vi "digital_demod_host_sp_step_height_fb.vi"() -> ()   [LabVIEW 2018]
uses:
  <vilib>/userdefined/High Color/nirio_resource_hc.ctl
  <vilib>/LabVIEW Targets/FPGA/RIO/nirio_PxiTriggers.ctl
  <vilib>/UPVI/lvhdf5/file.llb/LVH5F Operation.ctl
  <vilib>/UPVI/lvhdf5/dataset.llb/LVH5D Operation.ctl
  <vilib>/Utility/miscctls.llb/LVRectTypeDef.ctl
  <vilib>/UPVI/lvhdf5/group.llb/H5G_obj_t.ctl
  <vilib>/FPGAPlugInAG/PXI-7854R/niLvFpga_Open_PXI-7854R.vi
  <vilib>/rvi/interface/common/dynamic/niFpgaDynamicAddResources.vi
  <vilib>/FPGAPlugInAG/Dynamic/niLvFpga_Run_Dynamic.vi
  <vilib>/LabVIEW Targets/FPGA/RIO/nirioReserveTrigger.vi
  <vilib>/Utility/error.llb/Error Cluster From Error Code.vi
  <vilib>/rvi/errors/niLvFpgaAdjustHostInterfaceError.vi
  <vilib>/UPVI/lvhdf5/utility.llb/Select HDF5 Dialog.vi
  <vilib>/UPVI/lvhdf5/utility.llb/Select HDF5 Dialog (Object Only).vi
  <vilib>/UPVI/lvhdf5/dataset.llb/Simple H5Dwrite (Variant).vi
  <vilib>/FPGAPlugInAG/Dynamic/niLvFpga_Close_Dynamic.vi
  <vilib>/rvi/interface/nirviOpenFPGA/nirviOpenFPGA.xnode
  FPGA Bitfiles/digitaldemod_FPGATarget_digitaldemodfpga_GFAocKRMO-I.lvbitx
  <vilib>/rvi/interface/nirviMethod/nirviMethod.xnode
  <vilib>/rvi/interface/nirviReadWriteControl/nirviReadWriteControl.xnode
  <vilib>/UPVI/lvhdf5/dataset.llb/Simple H5Dwrite.xnode
  <vilib>/UPVI/lvhdf5/library.llb/HDF5 Ref.ctl
  <vilib>/rvi/interface/nirviCloseFPGA/nirviCloseFPGA.xnode
  <vilib>/rvi/interface/Simulation/niFpgaSimulationCallBeginRW.vi
  <vilib>/rvi/errors/niLvFpgaMergeErrorWithErrorCode.vi
  <vilib>/FPGAPlugInAG/Dynamic/niLvFpga_ReadFifo_Dynamic.vi
  NiFpgaLv.dll
  <vilib>/FPGAPlugInAG/Dynamic/niLvFpga_StartFifo_Dynamic.vi
  <vilib>/FPGAPlugInAG/Dynamic/niLvFpga_StopFifo_Dynamic.vi
  FPGA Timekeeper 1.1b0/FPGA Timekeeper.lvlib
  <vilib>/UPVI/lvhdf5/identifier.llb/Not an HDF5 Refnum Constant.vi
  <vilib>/UPVI/lvhdf5/dataset.llb/OpenCreateReplace Dataset by Element Type.vi
  <vilib>/UPVI/lvhdf5/dataspace.llb/H5Sselect_hyperslab.vi
  <vilib>/UPVI/lvhdf5/dataset.llb/H5Dwrite (Variant).vi
  <vilib>/UPVI/lvhdf5/dataset.llb/H5Dget_space.vi
  <vilib>/UPVI/lvhdf5/attribute.llb/private/LVH5AwriteWDTAttrs.vi
  <vilib>/UPVI/lvhdf5/dataspace.llb/H5Sclose.vi
  <vilib>/UPVI/lvhdf5/dataset.llb/H5Dclose.vi
  <vilib>/UPVI/lvhdf5/utility.llb/Select HDF5 Dialog (File and Object).vi
panel:
  in  "z_set_min":dbl=-920000.0
  in  "z_set_max":dbl=-850000.0
  out "current_z_set":dbl=-850500.0
  in  "step_lower_lim":dbl=-5000.0
  in  "step_upper_lim":dbl=5000.0
  out "height_fb":dbl=1600.0
  in  "height_pg":dbl=-10000.0
  in  "height_set_point":dbl=-0.8
  in  "Counts per update":i32=10000
  in  "Height_fb_counter":i32=7860
  in  "Height feedback":bool
  in  "Height_pcc":dbl=0.05
  in  "subtract_zfb_ndelay":u8=1
  in  "subtract_zfb_delay":bool=TRUE
  out "pow_fb":i16(graph)=-50
  in  "subtract_zfb_i_scale":fxp<+/-,32,16>=-17.0
  in  "subtract_zfb_p_scale":fxp<+/-,32,16>=-23.0
  in  "subtract_zfb_d_scale":fxp<+/-,32,16>=-13.0
  in  "subtract_zfb_from_powerr":bool=TRUE
  in  "sum_z-pow_fb":bool=TRUE
  in  "delta_pow_set_llim":fxp<+/-,32,32>=-80000.0
  in  "delta_pow_set_ulim":fxp<+/-,32,32>=80000.0
  in  "fb_on_powset":bool
  in  "pow_lower_lim":i16=-2000
  in  "pow_upper_lim":i16=2000
  in  "pow_dc_offset":i16=-17200
  in  "pow_dg":fxp<+/-,32,16>
  in  "pow_pg":fxp<+/-,32,16>
  in  "pow_fb":bool=TRUE
  out "pow_set_actual":fxp<+/-,33,33>=-34500.0
  in  "reset_pow_accum":bool
  in  "pow_bitshift":i16=-6
  in  "pow_fb_bitshift":i16=-16
  in  "pow_ig":fxp<+/-,32,16>=0.00140380859375
  in  "pow_set_user":fxp<+/-,32,32>=-34500.0
  out "pow":i32(graph)=-37680
  out "delta_pow_set":dbl(graph)
  in  "DAQ_trig":bool
  in  "save_data":bool=TRUE
  out "z_fb_tot":i16(graph)=-17096
  in  "z_off_restart":bool
  in  "z_off_step":i16=-17500
  in  "z_off_start":i16=-17500
  in  "step_z_offset":bool
  in  "z_set_step":fxp<+/-,32,32>
  in  "step_z_set":bool
  out "z_set_user":fxp<+/-,32,32>=-860000.0
  in  "set_z_init":bool
  in  "reset_zphi_and_change":bool
  in  "reset_z_accum":bool
  in  "z_lower_lim":i16=-3000
  in  "z_upper_lim":i16=3000
  in  "z_fb_bitshift":i16=-16
  in  "z_ig":fxp<+/-,32,16>=-1.52587890625e-05
  in  "z_dg":fxp<+/-,32,16>=-0.205291748046875
  in  "z_pg":fxp<+/-,32,16>=-0.010528564453125
  in  "z_bitshift":i16
  in  "z_set_init":fxp<+/-,32,32>=-860000.0
  in  "z_dc_offset":i16
  in  "z_internal_inject_scale":i16=400
  in  "z_internal_inject_freq":fxp<+,32,0>=2.00001522898674e-05 format="%#_32g"
  in  "add_sin":bool
  in  "show_quad":bool=TRUE
  out "delta_phi":cluster{dbl, dbl, dbl, dbl}(graph)={0.0, 0.05572509765625, 0.1119384765625, 0.0279541015625}
  in  "xy2_bitshift":i16
  in  "xy_fb_bitshift":i16=-16
  in  "y_lower_lim":i16=-1000
  in  "y_upper_lim":i16=1000
  in  "y_dg":fxp<+/-,32,16>=-0.004974365234375
  in  "x_lower_lim":i16=-1000
  in  "x_upper_lim":i16=1000
  in  "x_dg":fxp<+/-,32,16>=0.004974365234375
  in  "xy_bitshift":i16=-10
  in  "y_dc_offset":i16
  in  "x_dc_offset":i16
  in  "downsample->xyz":bool
  in  "inject_sigs":bool
  in  "Load last pars":bool
  out "config_trig":bool
  in  "block_hardware_trigs":bool
  out "config_loaded":bool
  out "Nsamp_config":u32=40000
  out "fpga_dat_path":path=path "D:/data/20210329/bead2/turbombar_powfb_xyzcool_1_fpga.h5"
  in  "reset_trigs":bool
  in  "accept_trigs":bool=TRUE
  out "amp4":dbl(graph)=9833.655883789062
  out "phi4":dbl(graph)=-66.42401123046875
  in  "Change Pars 2":bool
  out "z_fb":i16(graph)=154
  out "z":i32(graph)=-850000
  out "y_fb":i16(graph)=3
  out "y":i32(graph)=-88958
  out "x_fb":i16(graph)
  out "x":i32(graph)=-3908
  out "Host time (ns)":u64=1617643596633207808
  out "Target time (ns)":u64=1617643596633246868
  in  "downsamp_num":i16=100
  in  "Reset Phi Params":T1={"All Phi?"=FALSE, "Which?"=enum."3"}
  out "amp2":dbl(graph)=4850.323699951172
  out "amp3":dbl(graph)=5487.453506469727
  out "amp0":dbl(graph)=5014.9466552734375
  out "amp1":dbl(graph)=5412.640853881836
  out "phi2":dbl(graph)=-6.08233642578125
  out "phi3":dbl(graph)=-6.16632080078125
  in  "subtract_mean":bool=TRUE
  out "loop time":fxp<+,32,32>=2.0
  in  "Change Pars":bool
  out "phi0":dbl(graph)=-6.19427490234375
  out "phi1":dbl(graph)=-6.1385498046875
  in  "counter offset":u32
  in  "phase discont_neg":fxp<+/-,24,12>=-1.0
  in  "phase discont_pos":fxp<+/-,24,12>=1.0
  in  "Reset Phi":bool
  in  "loop timer (usec)":u32=2
  in  "Update ADC Clock":bool
  in  "Host Update Rate (msec)":dbl=1.0 format="%#_13g"
  in  "RIO Device":T2="RIO0"
  # "QPD AMPLITUDES"
  # "QPD PHASES"
  # "BACKSCATTER"
  # "BEAD XYZ + FB"
  # "FEEDBACK NESTING"
  # "Height feedback"
  # "POWER FEEDBACK"
  # "Z FEEDBACK"
  # "X FEEDBACK"
  # "Y FEEDBACK"
types:
  T1 = cluster{"All Phi?":bool, "Which?":enum16{"0", "1", "2", "3", "4"}}
  T2 = typedef "nirio_resource_hc.ctl" = tag
  T3 = typedef "nirio_PxiTriggers.ctl" = u16
  T4 = cluster{"phase discont_pos":fxp<+/-,24,12>, "phase discont_neg":fxp<+/-,24,12>, "counter offset":u32, "subtract_mean":bool, "downsamp_num":i16, "xy_bitshift":i16, "x_dg":fxp<+/-,32,16>, "x_upper_lim":i16, "x_lower_lim":i16, "x_dc_offset":i16, "y_dg":fxp<+/-,32,16>, "y_upper_lim":i16, "y_lower_lim":i16, "y_dc_offset":i16, "xy_fb_bitshift":i16, "z_bitshift":i16, "z_set_init":fxp<+/-,32,32>, "z_pg":fxp<+/-,32,16>, "z_dg":fxp<+/-,32,16>, "z_ig":fxp<+/-,32,16>, "z_fb_bitshift":i16, "z_upper_lim":i16, "z_lower_lim":i16, "z_off_start":i16, "inject_sigs":bool, "downsample->xyz":bool, "xy2_bitshift":i16, "add_sin":bool, "z_internal_inject_freq":fxp<+,32,0>, "z_internal_inject_scale":i16, "pow_bitshift":i16, "pow_set_user":fxp<+/-,32,32>, "pow_pg":fxp<+/-,32,16>, "pow_dg":fxp<+/-,32,16>, "pow_ig":fxp<+/-,32,16>, "pow_dc_offset":i16, "pow_upper_lim":i16, "pow_lower_lim":i16, "pow_fb_bitshift":i16, "pow_fb":bool, "fb_on_powset":bool, "delta_pow_set_ulim":fxp<+/-,32,32>, "delta_pow_set_llim":fxp<+/-,32,32>, "sum_z-pow_fb":bool, "subtract_zfb_from_powerr":bool, "subtract_zfb_p_scale":fxp<+/-,32,16>, "subtract_zfb_i_scale":fxp<+/-,32,16>, "subtract_zfb_d_scale":fxp<+/-,32,16>, "subtract_zfb_delay":bool, "subtract_zfb_ndelay":u8}
  T5 = enum16{"open", "replace", "create", "open or create", "replace or create", "replace or create with confirmation"}
  T6 = typedef "LVH5F Operation.ctl" = enum16{"open", "open or create", "create or replace", "create or replace (with confirmation)", "create", "open (read only)"}
  T7 = typedef "LVRectTypeDef.ctl" = cluster{"Left":i16, "Top":i16, "Right":i16, "Bottom":i16}
  T8 = cluster{"Behavior":enum32{"Invalid", "Default", "Floating", "Floating/Auto-Hide", "Modal"}, "Position":T7, "Center":bool, "Title":string}
  T9 = typedef "LVH5D Operation.ctl" = enum16{"open", "replace", "create", "open or create", "create or replace", "create or replace with confirmation"}
  T10 = typedef "H5G_obj_t.ctl" = i32
  T11 = cluster{"Object Types (any)":T10[], "Object Pattern":string}
  T12 = typedef "HDF5 Ref.ctl" = refnum<k1>
  T13 = cluster{fxp<+/-,33,19>, fxp<+/-,33,19>, fxp<+/-,33,19>, fxp<+/-,33,19>}
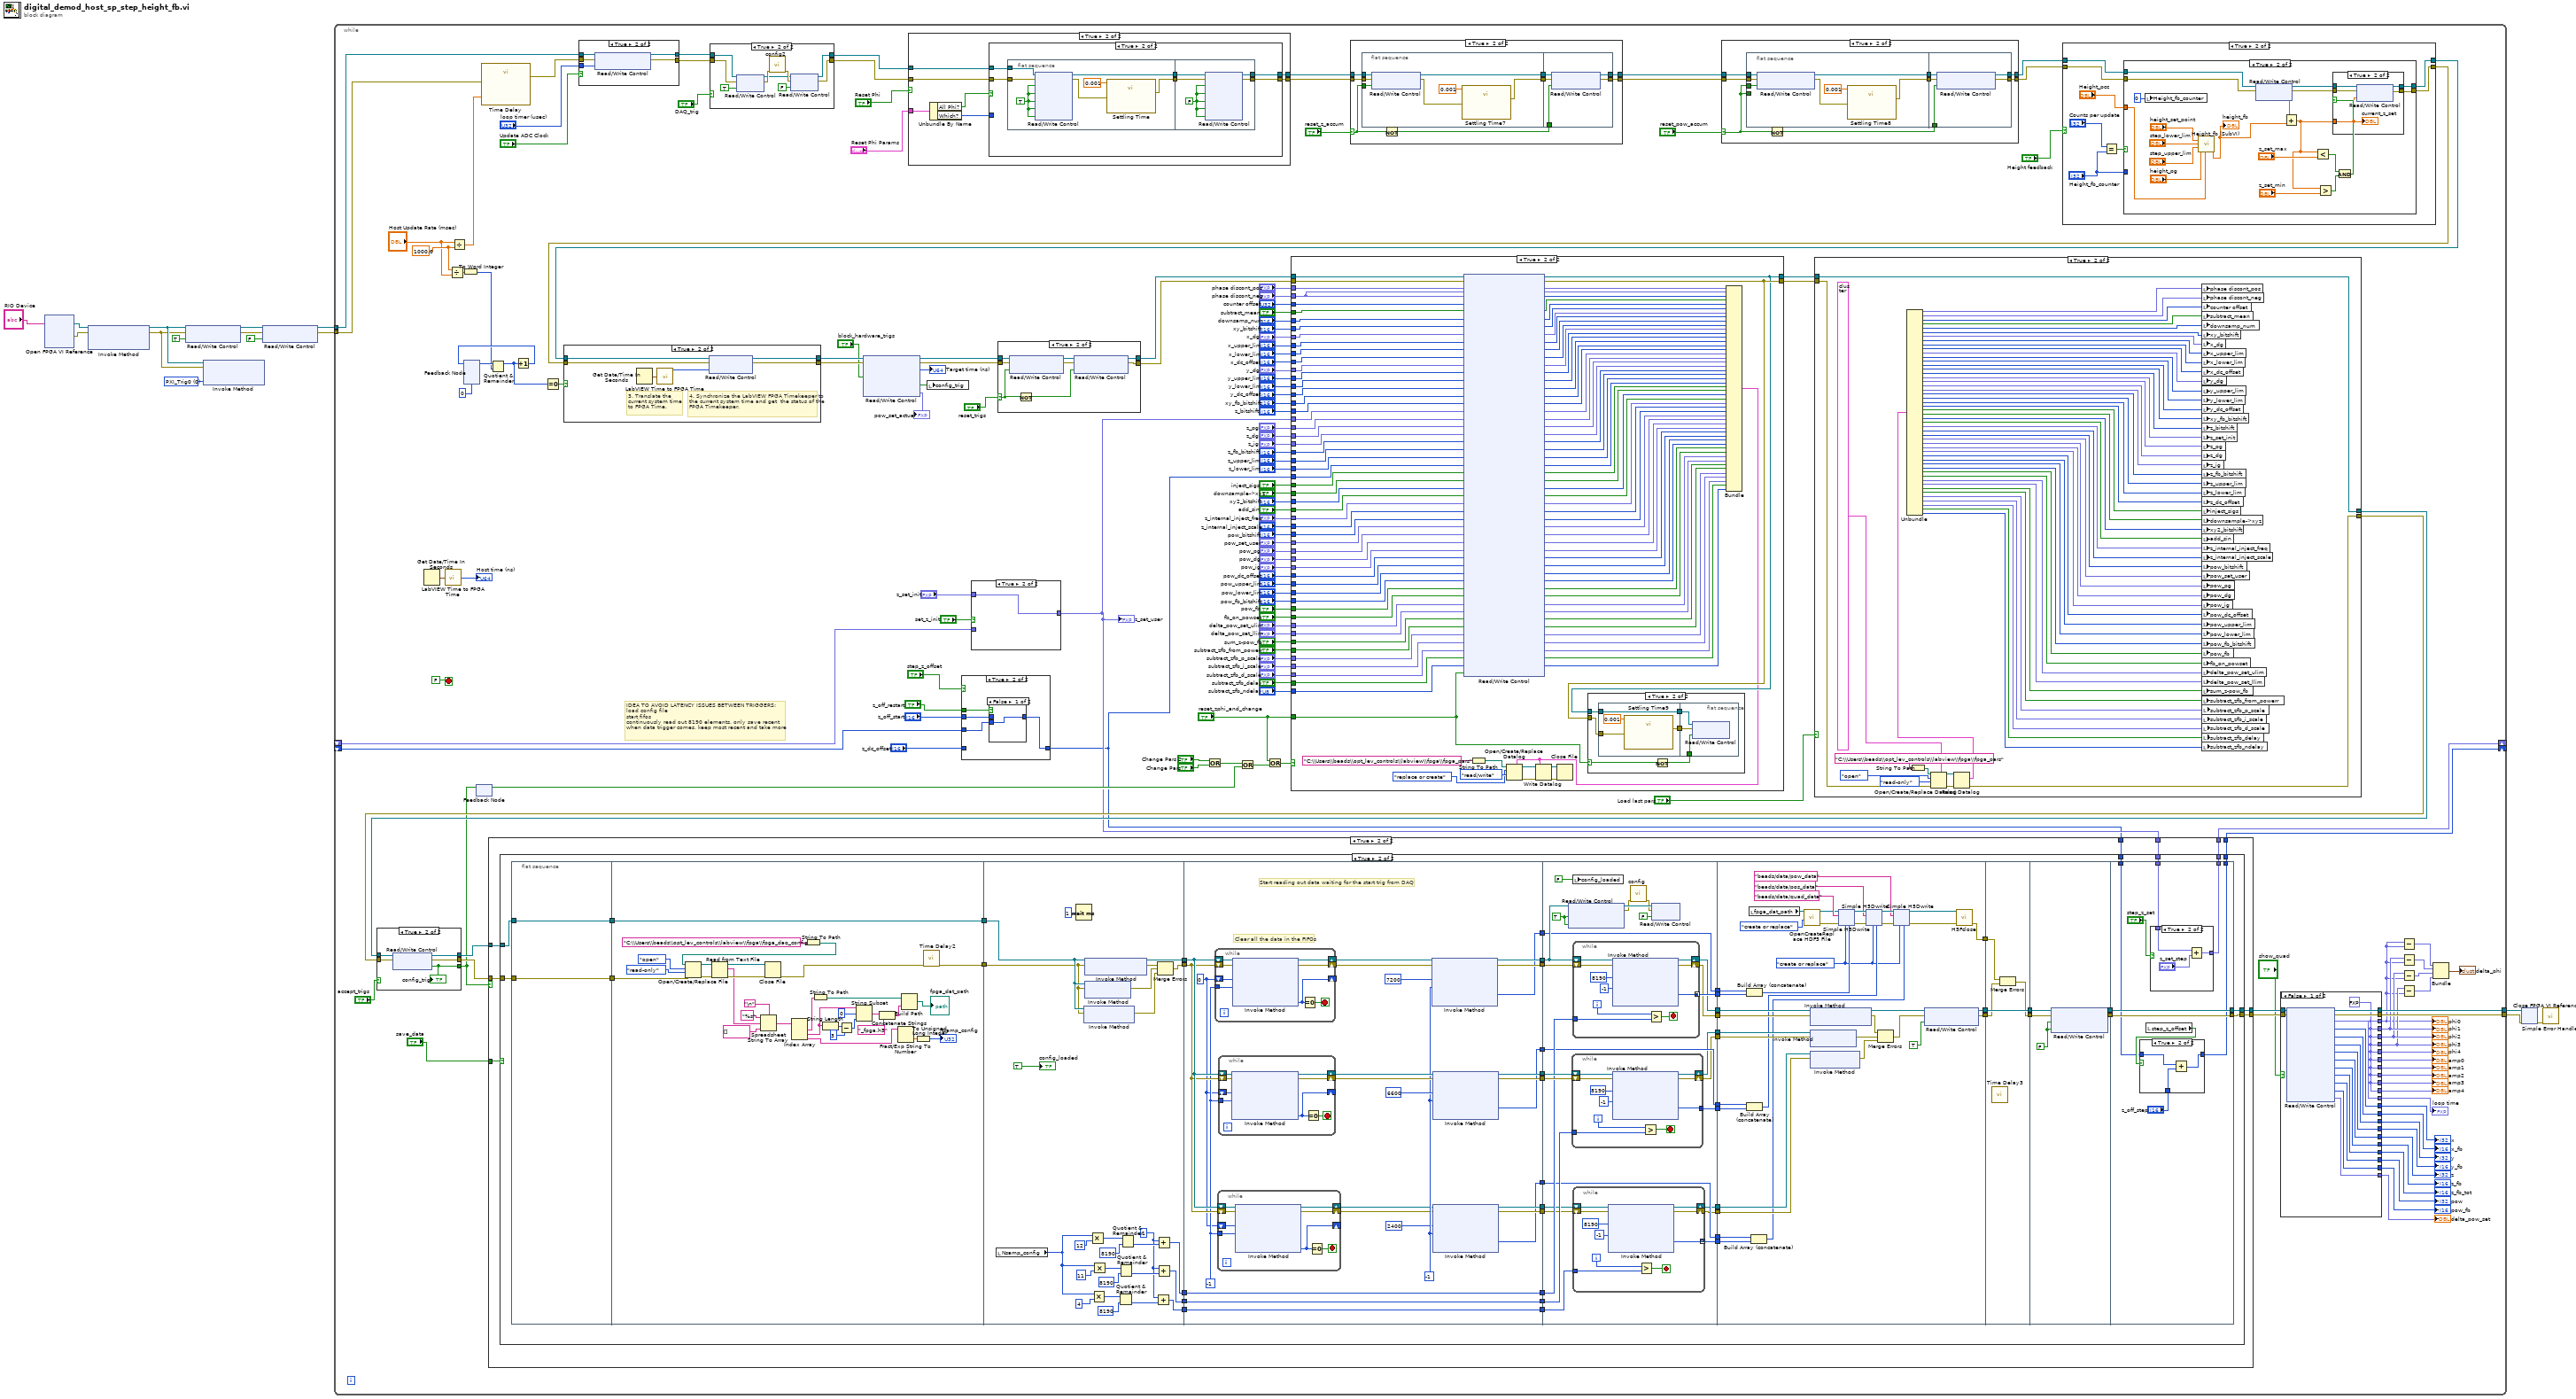
[diagram p0: block diagram]
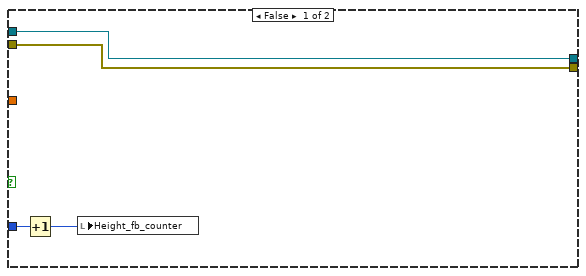
[diagram p3: hidden frame]
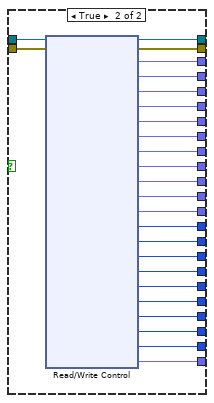
[diagram p10: hidden frame]
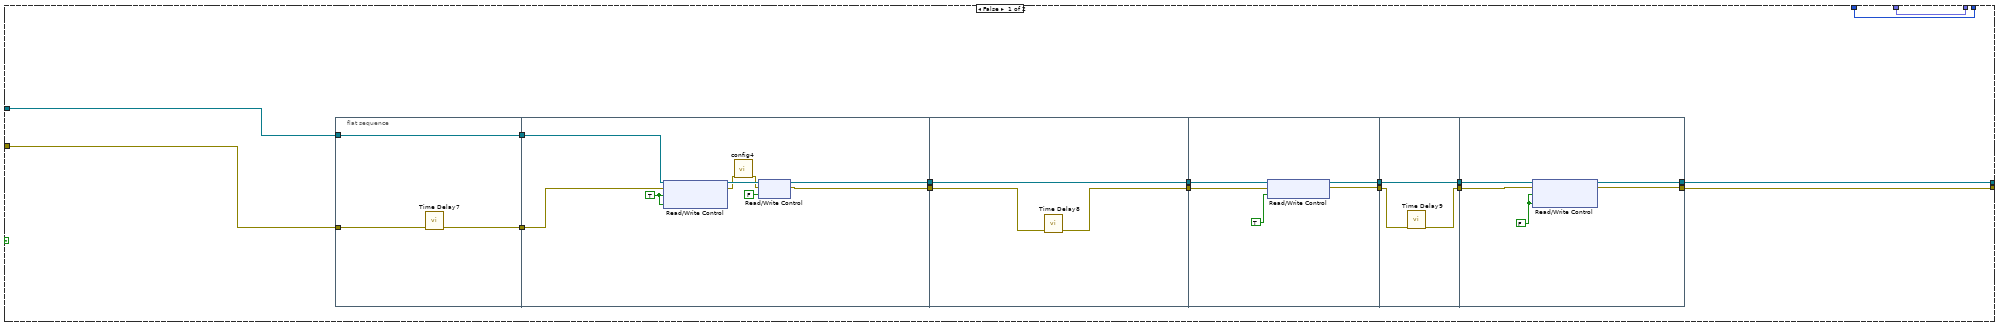
[diagram p15: hidden frame]
diagram:
  w1 = T3 0 items=["PXI_Trig0", "PXI_Trig1", "PXI_Trig2", "PXI_Trig3", "PXI_Trig4", "PXI_Trig5", "PXI_Trig6", "PXI_Trig7"] ("Trigger")
  n1 = xnode "Open FPGA VI Reference"("resource name"="RIO Device") -> ("FPGA VI Reference Out"=w11:refnum<k20>, "error out"=w10:errorcluster)  [unwired: 1 in]
  n2 = xnode "Invoke Method"("FPGA VI Reference In"=w11, "error in"=w10) -> ("FPGA VI Reference Out"=w3:refnum<k20>, "error out"=w2:errorcluster)  [unwired: 1 in]
  n3 = xnode "Read/Write Control"("FPGA VI Reference In"=w3, "error in"=w2, "reset_config_trig"=TRUE ("reset_trig")) -> ("FPGA VI Reference Out"=w6:refnum<k20>, "error out"=w4:errorcluster)
  n4 = xnode "Invoke Method"("FPGA VI Reference In"=w3, "error in"=w2, "Trigger"=w1) -> ()  [unwired: 2 out]
  n5 = xnode "Read/Write Control"("FPGA VI Reference In"=w6, "error in"=w4, "reset_config_trig"=FALSE ("manual_trig")) -> ("FPGA VI Reference Out"=w9:refnum<k20>, "error out"=w8:errorcluster)
  n6 = while {
    tunnel: w8 -> [w169]
    tunnel: w9 -> [w95]
    tunnel: [w162] -> w14
    tunnel: [w161] -> w13
    shift-right: [w73] -> _
    shift-left: _ -> [w74]
    shift-right: [w65] -> _
    shift-left: _ -> [w64]
    stop <- FALSE stop-if-true
    w152 = 1000.0
    # "IDEA TO AVOID LATENCY ISSUES BETWEEN TRIGGERS:\nload config file\nstart fifos\ncontinuously read out 8190 elements, only save recent\nwhen data trigger comes, keep most recent and take more"
    n7 = Get Date/Time In Seconds() -> (seconds since 1Jan1904=w141:timestamp)
    n8 = call "LabVIEW Time to FPGA Time.vi"("LabVIEW time"=w141) -> ("FPGA time (ns)"=→"Host time (ns)":u64)
    n9 = Divide(x=w152, y="Host Update Rate (msec)") -> (x/y=w150:dbl)
    n10 = Divide(x="Host Update Rate (msec)", y=w152) -> (x/y=w170:dbl)
    n11 = To Word Integer(number=w150) -> (16bit integer=w144:i16)
    n12 = feedback #1(i16 0) -> (w146:i16)
    n13 = feedback #2() -> (w76:bool)  [unwired: 1 in]
    n14 = call "Time Delay"("error in (no error)"=w169, "Delay Time (s)"=w170) -> ("error out"=w167:errorcluster)  [unwired: 9 in]
    n15 = Quotient & Remainder(x=w146, y=w144) -> (x-y*floor(x/y)=w143:i16)  [unwired: 1 out]
    n16 = Increment(x=w143) -> (x+1=w145:i16)
    n17 = feedback-in #1(w145) -> ()
    n18 = Equal To 0?(x=w143) -> (x = 0?=w148:bool)
    n19 = case shown="True" "Update ADC Clock" {
      tunnel: w95 -> [w1549 w1554]
      tunnel: w167 -> [w1548 w1553]
      tunnel: [w1549 w1552] -> w53
      tunnel: [w1548 w1551] -> w52
      tunnel: "loop timer (usec)" -> [_ w1550]
      frame False {
      }
      frame True {
        n20 = xnode "Read/Write Control"("FPGA VI Reference In"=w1554, "error in"=w1553, "loop timer (usec)"=w1550) -> ("FPGA VI Reference Out"=w1552:refnum<k20>, "error out"=w1551:errorcluster)
      }
    }
    n21 = case shown="True" "DAQ_trig" {
      tunnel: w53 -> [w235 w239]
      tunnel: w52 -> [w234 w238]
      tunnel: [w235 w237] -> w51
      tunnel: [w234 w236] -> w50
      frame False {
      }
      frame True {
        n22 = xnode "Read/Write Control"("FPGA VI Reference In"=w239, "error in"=w238, "TRIG0"=TRUE) -> ("FPGA VI Reference Out"=w241:refnum<k20>, "error out"=w242:errorcluster)
        n23 = call "config2"("error in (no error)"=w242) -> ("error out"=w243:errorcluster)  [unwired: 10 in]
        n24 = xnode "Read/Write Control"("FPGA VI Reference In"=w241, "error in"=w243, "TRIG0"=FALSE) -> ("FPGA VI Reference Out"=w237:refnum<k20>, "error out"=w236:errorcluster)
      }
    }
    n25 = case shown="True" "Reset Phi" {
      tunnel: w51 -> [w1427 w1434]
      tunnel: w50 -> [w1426 w1433]
      tunnel: [w1427 w1431] -> w99
      tunnel: [w1426 w1432] -> w98
      tunnel: "Reset Phi Params" -> [_ w1430]
      frame False {
      }
      frame True {
        n26 = Unbundle By Name(w1430) -> ("All Phi?"=w1429:bool, "Which?"=w1428:enum16{"0", "1", "2", "3", "4"})
        n27 = case shown="True" w1429 {
          tunnel: w1434 -> [w1439 w1533]
          tunnel: w1433 -> [w1438 w1532]
          tunnel: [w1436 w1531] -> w1432
          tunnel: [w1437 w1530] -> w1431
          tunnel: w1428 -> [w1435 _]
          frame False {
            n28 = case shown="\"4\"" w1435 {
              tunnel: w1439 -> [w1443 w1461 w1479 w1497 w1515]
              tunnel: w1438 -> [w1442 w1460 w1478 w1496 w1514]
              tunnel: [w1441 w1459 w1477 w1495 w1513] -> w1437
              tunnel: [w1440 w1458 w1476 w1494 w1512] -> w1436
              frame "1" {
                n29 = flat-sequence {
                  tunnel: w1443 -> [w1452]
                  tunnel: w1442 -> [w1451]
                  tunnel: [w1450] -> w1445
                  tunnel: [w1447] -> w1444
                  tunnel: w1445 -> [w1457]
                  tunnel: w1444 -> [w1456]
                  tunnel: [w1455] -> w1441
                  tunnel: [w1454] -> w1440
                  frame #0 {
                    n30 = xnode "Read/Write Control"("FPGA VI Reference In"=w1452, "error in"=w1451, "reset_phi1"=TRUE) -> ("FPGA VI Reference Out"=w1450:refnum<k20>, "error out"=w1448:errorcluster)
                    n31 = call "Settling Time2"("error in (no error)"=w1448, "Delay Time (s)"=0.001) -> ("error out"=w1447:errorcluster)  [unwired: 9 in]
                  }
                  frame #1 {
                    n32 = xnode "Read/Write Control"("FPGA VI Reference In"=w1457, "error in"=w1456, "reset_phi1"=FALSE) -> ("FPGA VI Reference Out"=w1455:refnum<k20>, "error out"=w1454:errorcluster)
                  }
                }
              }
              frame "2" {
                n33 = flat-sequence {
                  tunnel: w1461 -> [w1470]
                  tunnel: w1460 -> [w1469]
                  tunnel: [w1468] -> w1463
                  tunnel: [w1465] -> w1462
                  tunnel: w1463 -> [w1475]
                  tunnel: w1462 -> [w1474]
                  tunnel: [w1473] -> w1459
                  tunnel: [w1472] -> w1458
                  frame #0 {
                    n34 = xnode "Read/Write Control"("FPGA VI Reference In"=w1470, "error in"=w1469, "reset_phi2"=TRUE) -> ("FPGA VI Reference Out"=w1468:refnum<k20>, "error out"=w1466:errorcluster)
                    n35 = call "Settling Time3"("error in (no error)"=w1466, "Delay Time (s)"=0.001) -> ("error out"=w1465:errorcluster)  [unwired: 9 in]
                  }
                  frame #1 {
                    n36 = xnode "Read/Write Control"("FPGA VI Reference In"=w1475, "error in"=w1474, "reset_phi2"=FALSE) -> ("FPGA VI Reference Out"=w1473:refnum<k20>, "error out"=w1472:errorcluster)
                  }
                }
              }
              frame "3" {
                n37 = flat-sequence {
                  tunnel: w1479 -> [w1488]
                  tunnel: w1478 -> [w1487]
                  tunnel: [w1486] -> w1481
                  tunnel: [w1483] -> w1480
                  tunnel: w1481 -> [w1493]
                  tunnel: w1480 -> [w1492]
                  tunnel: [w1491] -> w1477
                  tunnel: [w1490] -> w1476
                  frame #0 {
                    n38 = xnode "Read/Write Control"("FPGA VI Reference In"=w1488, "error in"=w1487, "reset_phi3"=TRUE) -> ("FPGA VI Reference Out"=w1486:refnum<k20>, "error out"=w1484:errorcluster)
                    n39 = call "Settling Time4"("error in (no error)"=w1484, "Delay Time (s)"=0.001) -> ("error out"=w1483:errorcluster)  [unwired: 9 in]
                  }
                  frame #1 {
                    n40 = xnode "Read/Write Control"("FPGA VI Reference In"=w1493, "error in"=w1492, "reset_phi3"=FALSE) -> ("FPGA VI Reference Out"=w1491:refnum<k20>, "error out"=w1490:errorcluster)
                  }
                }
              }
              frame "4" {
                n41 = flat-sequence {
                  tunnel: w1497 -> [w1506]
                  tunnel: w1496 -> [w1505]
                  tunnel: [w1504] -> w1499
                  tunnel: [w1501] -> w1498
                  tunnel: w1499 -> [w1511]
                  tunnel: w1498 -> [w1510]
                  tunnel: [w1509] -> w1495
                  tunnel: [w1508] -> w1494
                  frame #0 {
                    n42 = xnode "Read/Write Control"("FPGA VI Reference In"=w1506, "error in"=w1505, "reset_phi4"=TRUE) -> ("FPGA VI Reference Out"=w1504:refnum<k20>, "error out"=w1502:errorcluster)
                    n43 = call "Settling Time5"("error in (no error)"=w1502, "Delay Time (s)"=0.001) -> ("error out"=w1501:errorcluster)  [unwired: 9 in]
                  }
                  frame #1 {
                    n44 = xnode "Read/Write Control"("FPGA VI Reference In"=w1511, "error in"=w1510, "reset_phi4"=FALSE) -> ("FPGA VI Reference Out"=w1509:refnum<k20>, "error out"=w1508:errorcluster)
                  }
                }
              }
              frame "0" {
                n45 = flat-sequence {
                  tunnel: w1515 -> [w1524]
                  tunnel: w1514 -> [w1523]
                  tunnel: [w1522] -> w1517
                  tunnel: [w1519] -> w1516
                  tunnel: w1517 -> [w1529]
                  tunnel: w1516 -> [w1528]
                  tunnel: [w1527] -> w1513
                  tunnel: [w1526] -> w1512
                  frame #0 {
                    n46 = xnode "Read/Write Control"("FPGA VI Reference In"=w1524, "error in"=w1523, "reset_phi0"=TRUE) -> ("FPGA VI Reference Out"=w1522:refnum<k20>, "error out"=w1520:errorcluster)
                    n47 = call "Settling Time6"("error in (no error)"=w1520, "Delay Time (s)"=0.001) -> ("error out"=w1519:errorcluster)  [unwired: 9 in]
                  }
                  frame #1 {
                    n48 = xnode "Read/Write Control"("FPGA VI Reference In"=w1529, "error in"=w1528, "reset_phi0"=FALSE) -> ("FPGA VI Reference Out"=w1527:refnum<k20>, "error out"=w1526:errorcluster)
                  }
                }
              }
            }
          }
          frame True {
            n49 = flat-sequence {
              tunnel: w1533 -> [w1542]
              tunnel: w1532 -> [w1541]
              tunnel: [w1540] -> w1535
              tunnel: [w1537] -> w1534
              tunnel: w1535 -> [w1547]
              tunnel: w1534 -> [w1546]
              tunnel: [w1545] -> w1530
              tunnel: [w1544] -> w1531
              frame #0 {
                w1536 = TRUE
                n50 = xnode "Read/Write Control"("FPGA VI Reference In"=w1542, "error in"=w1541, "reset_phi0"=w1536, "reset_phi1"=w1536, "reset_phi2"=w1536, "reset_phi3"=w1536, "reset_phi4"=w1536) -> ("FPGA VI Reference Out"=w1540:refnum<k20>, "error out"=w1538:errorcluster)
                n51 = call "Settling Time"("error in (no error)"=w1538, "Delay Time (s)"=0.001) -> ("error out"=w1537:errorcluster)  [unwired: 9 in]
              }
              frame #1 {
                w1543 = FALSE
                n52 = xnode "Read/Write Control"("FPGA VI Reference In"=w1547, "error in"=w1546, "reset_phi0"=w1543, "reset_phi1"=w1543, "reset_phi2"=w1543, "reset_phi3"=w1543, "reset_phi4"=w1543) -> ("FPGA VI Reference Out"=w1545:refnum<k20>, "error out"=w1544:errorcluster)
              }
            }
          }
        }
      }
    }
    n53 = case shown="True" "step_z_offset" {
      tunnel: [w245 w246] -> w66
      tunnel: "z_dc_offset" -> [w245 _]
      tunnel: w64 -> [_ w248]
      tunnel: "z_off_start" -> [_ w249]
      tunnel: "z_off_restart" -> [_ w247]
      frame False {
      }
      frame True {
        n54 = case shown="False" w247 {
          tunnel: w249 -> [_ w251]
          tunnel: w248 -> [w250 _]
          tunnel: [w250 w251] -> w246
          frame False {
          }
          frame True {
          }
        }
      }
    }
    n55 = case shown="True" "set_z_init" {
      tunnel: [w252 w253] -> w72
      tunnel: "z_set_init" -> [_ w253]
      tunnel: w74 -> [w252 _]
      frame False {
      }
      frame True {
      }
    }
    "z_set_user" <- w72
    n56 = Or(x="Change Pars 2", y="Change Pars") -> (x .or. y?=w29:bool)
    n57 = Or(x=w29, y=w76) -> (x .or. y?=w27:bool)
    n58 = Or(x="reset_zphi_and_change", y=w27) -> (x .or. y?=w26:bool)
    n59 = case shown="True" "reset_z_accum" {
      selector: "reset_z_accum" -> [_ w361]
      tunnel: w99 -> [w359 w367]
      tunnel: w98 -> [w358 w366]
      tunnel: [w359 w365] -> w49
      tunnel: [w358 w364] -> w48
      frame False {
      }
      frame True {
        n60 = flat-sequence {
          tunnel: w367 -> [w374]
          tunnel: w366 -> [w373]
          tunnel: w361 -> [w371]
          tunnel: [w372] -> w363
          tunnel: [w368] -> w362
          tunnel: [w376] -> w364
          tunnel: [w377] -> w365
          tunnel: w363 -> [w379]
          tunnel: w362 -> [w378]
          tunnel: w360 -> [w375]
          frame #0 {
            n61 = xnode "Read/Write Control"("FPGA VI Reference In"=w374, "error in"=w373, "reset_z_accum"=w371) -> ("FPGA VI Reference Out"=w372:refnum<k20>, "error out"=w369:errorcluster)
            n62 = call "Settling Time7"("error in (no error)"=w369, "Delay Time (s)"=0.001) -> ("error out"=w368:errorcluster)  [unwired: 9 in]
          }
          frame #1 {
            n63 = xnode "Read/Write Control"("FPGA VI Reference In"=w379, "error in"=w378, "reset_z_accum"=w375) -> ("FPGA VI Reference Out"=w377:refnum<k20>, "error out"=w376:errorcluster)
          }
        }
        n64 = Not(x=w361) -> (.not. x?=w360:bool)
      }
    }
    n65 = case shown="True" "reset_pow_accum" {
      selector: "reset_pow_accum" -> [_ w216]
      tunnel: w49 -> [w213 w218]
      tunnel: w48 -> [w212 w217]
      tunnel: [w213 w215] -> w19
      tunnel: [w212 w214] -> w17
      frame False {
      }
      frame True {
        n66 = flat-sequence {
          tunnel: w218 -> [w228]
          tunnel: w217 -> [w227]
          tunnel: w216 -> [w225]
          tunnel: [w226] -> w221
          tunnel: [w222] -> w220
          tunnel: w216 -> [_]
          tunnel: [w229] -> _
          tunnel: [w231] -> w215
          tunnel: w221 -> [w233]
          tunnel: w220 -> [w232]
          tunnel: w219 -> [w230]
          tunnel: [w229] -> w214
          frame #0 {
            n67 = xnode "Read/Write Control"("FPGA VI Reference In"=w228, "error in"=w227, "reset_pow_accum"=w225) -> ("FPGA VI Reference Out"=w226:refnum<k20>, "error out"=w223:errorcluster)
            n68 = call "Settling Time8"("error in (no error)"=w223, "Delay Time (s)"=0.001) -> ("error out"=w222:errorcluster)  [unwired: 9 in]
          }
          frame #1 {
            n69 = xnode "Read/Write Control"("FPGA VI Reference In"=w233, "error in"=w232, "reset_pow_accum"=w230) -> ("FPGA VI Reference Out"=w231:refnum<k20>, "error out"=w229:errorcluster)
          }
        }
        n70 = Not(x=w216) -> (.not. x?=w219:bool)
      }
    }
    n71 = case shown="True" "Height feedback" {
      tunnel: w19 -> [w172 w175]
      tunnel: [w172 w173] -> w18
      tunnel: w17 -> [w171 w176]
      tunnel: [w171 w174] -> w16
      frame False {
      }
      frame True {
        n72 = Equal?(x="Counts per update", y="Height_fb_counter") -> (x = y?=w180:bool)
        n73 = case shown="True" w180 {
          tunnel: "Height_fb_counter" -> [w183 _]
          tunnel: "Height_pcc" -> [_ w203]
          tunnel: w176 -> [w181 w197]
          tunnel: w175 -> [w182 w198]
          tunnel: [w181 w196] -> w174
          tunnel: [w182 w195] -> w173
          frame False {
            n74 = Increment(x=w183) -> (x+1=w184:i32)
            n75 = local write "Height_fb_counter"(w184) -> ()
          }
          frame True {
            n76 = local write "Height_fb_counter"(0 ("Height_fb_counter")) -> ()
            n77 = call "Height_fb (SubVI).vi"("Height_pcc"=w203, "height_set_point"="height_set_point", "height_pg"="height_pg", "step_upper_lim"="step_upper_lim", "step_lower_lim"="step_lower_lim") -> ("hieght_fb_out"=w191:dbl)  [unwired: 5 in, 1 out]
            "height_fb" <- w191
            n78 = xnode "Read/Write Control"("FPGA VI Reference In"=w198, "error in"=w197) -> ("FPGA VI Reference Out"=w194:refnum<k20>, "error out"=w193:errorcluster, "z_set_user"=w192:fxp<+/-,32,32>)
            n79 = Add(x=w192, y=w191) -> (x+y=w186:dbl)
            n80 = Less?(x=w186, y="z_set_max") -> (x < y?=w187:bool)
            n81 = Greater?(x=w186, y="z_set_min") -> (0:w188:bool)
            n82 = And(x=w187, y=w188) -> (x .and. y?=w185:bool)
            n83 = case shown="True" w185 {
              tunnel: [w205 w211] -> w196
              tunnel: [w206 w210] -> w195
              tunnel: w194 -> [w206 w209]
              tunnel: w193 -> [w205 w208]
              tunnel: w186 -> [_ w207]
              frame False {
              }
              frame True {
                n84 = xnode "Read/Write Control"("FPGA VI Reference In"=w209, "error in"=w208, "z_set_user"=w207) -> ("FPGA VI Reference Out"=w210:refnum<k20>, "error out"=w211:errorcluster)
                "current_z_set" <- w207
              }
            }
          }
        }
      }
    }
    n85 = case shown="True" w148 {
      tunnel: w16 -> [w1339 w1344]
      tunnel: w18 -> [w1340 w1343]
      tunnel: [w1340 w1342] -> w139
      tunnel: [w1339 w1341] -> w138
      frame False {
      }
      frame True {
        # "4. Synchronize the LabVIEW FPGA Timekeeper to the current system time and get  the status of the FPGA Timekeeper."
        # "3. Translate the current system time to FPGA Time."
        n86 = Get Date/Time In Seconds() -> (seconds since 1Jan1904=w1346:timestamp)
        n87 = call "LabVIEW Time to FPGA Time.vi"("LabVIEW time"=w1346) -> ("FPGA time (ns)"=w1345:u64)
        n88 = xnode "Read/Write Control"("FPGA VI Reference In"=w1343, "error in"=w1344, "RT time (ns)"=w1345) -> ("FPGA VI Reference Out"=w1342:refnum<k20>, "error out"=w1341:errorcluster)
      }
    }
    n89 = xnode "Read/Write Control"("FPGA VI Reference In"=w139, "error in"=w138, "block_config_trig"="block_hardware_trigs") -> ("FPGA VI Reference Out"=w110:refnum<k20>, "error out"=w109:errorcluster, "time (ns)"=→"Target time (ns)":u64, "config_trig"=w96:bool, "pow_set_actual"=→"pow_set_actual":fxp<+/-,33,33>)
    n90 = local write "config_trig"(w96) -> ()
    n91 = case shown="True" "reset_trigs" {
      selector: "reset_trigs" -> [_ w1332]
      tunnel: w110 -> [w1330 w1338]
      tunnel: w109 -> [w1329 w1337]
      tunnel: [w1330 w1334] -> w106
      tunnel: [w1329 w1333] -> w105
      frame False {
      }
      frame True {
        n92 = xnode "Read/Write Control"("FPGA VI Reference In"=w1338, "error in"=w1337, "reset_config_trig"=w1332) -> ("FPGA VI Reference Out"=w1336:refnum<k20>, "error out"=w1335:errorcluster)
        n93 = Not(x=w1332) -> (.not. x?=w1331:bool)
        n94 = xnode "Read/Write Control"("FPGA VI Reference In"=w1336, "error in"=w1335, "reset_config_trig"=w1331) -> ("FPGA VI Reference Out"=w1334:refnum<k20>, "error out"=w1333:errorcluster)
      }
    }
    n95 = case shown="True" w26 {
      tunnel: w105 -> [w1348 w1411]
      tunnel: [w1348 w1354] -> w92
      tunnel: [w1347 w1353] -> w94
      tunnel: w106 -> [w1347 w1412]
      tunnel: "phase discont_pos" -> [_ w1410]
      tunnel: "phase discont_neg" -> [_ w1409]
      tunnel: "counter offset" -> [_ w1408]
      tunnel: "subtract_mean" -> [_ w1407]
      tunnel: "downsamp_num" -> [_ w1406]
      tunnel: "x_dc_offset" -> [_ w1401]
      tunnel: "y_dc_offset" -> [_ w1397]
      tunnel: w66 -> [_ w1387]
      tunnel: w72 -> [_ w1394]
      tunnel: "xy_bitshift" -> [_ w1405]
      tunnel: "x_dg" -> [_ w1404]
      tunnel: "x_upper_lim" -> [_ w1403]
      tunnel: "x_lower_lim" -> [_ w1402]
      tunnel: "y_dg" -> [_ w1400]
      tunnel: "y_upper_lim" -> [_ w1399]
      tunnel: "y_lower_lim" -> [_ w1398]
      tunnel: "z_bitshift" -> [_ w1395]
      tunnel: "z_pg" -> [_ w1393]
      tunnel: "z_dg" -> [_ w1392]
      tunnel: "z_ig" -> [_ w1391]
      tunnel: "z_fb_bitshift" -> [_ w1390]
      tunnel: "z_upper_lim" -> [_ w1389]
      tunnel: "z_lower_lim" -> [_ w1388]
      tunnel: "xy_fb_bitshift" -> [_ w1396]
      tunnel: "inject_sigs" -> [_ w1378]
      tunnel: "downsample->xyz" -> [_ w1377]
      tunnel: "xy2_bitshift" -> [_ w1376]
      tunnel: "add_sin" -> [_ w1375]
      tunnel: "z_internal_inject_freq" -> [_ w1374]
      tunnel: "z_internal_inject_scale" -> [_ w1373]
      tunnel: "pow_set_user" -> [_ w1371]
      tunnel: "pow_ig" -> [_ w1370]
      tunnel: "pow_fb_bitshift" -> [_ w1364]
      tunnel: "pow_bitshift" -> [_ w1372]
      tunnel: "fb_on_powset" -> [_ w1362]
      tunnel: "delta_pow_set_ulim" -> [_ w1361]
      tunnel: "delta_pow_set_llim" -> [_ w1360]
      tunnel: "pow_fb" -> [_ w1363]
      tunnel: "pow_pg" -> [_ w1368]
      tunnel: "pow_dg" -> [_ w1369]
      tunnel: "pow_dc_offset" -> [_ w1367]
      tunnel: "pow_upper_lim" -> [_ w1366]
      tunnel: "pow_lower_lim" -> [_ w1365]
      tunnel: "sum_z-pow_fb" -> [_ w1359]
      tunnel: "subtract_zfb_from_powerr" -> [_ w1358]
      tunnel: "subtract_zfb_d_scale" -> [_ w1357]
      tunnel: "subtract_zfb_p_scale" -> [_ w1356]
      tunnel: "subtract_zfb_i_scale" -> [_ w1355]
      tunnel: "reset_zphi_and_change" -> [_ w1351]
      tunnel: "subtract_zfb_delay" -> [_ w1350]
      tunnel: "subtract_zfb_ndelay" -> [_ w1349]
      frame False {
      }
      frame True {
        n96 = xnode "Read/Write Control"("FPGA VI Reference In"=w1412, "error in"=w1411, "discont_pos"=w1410, "discont_neg"=w1409, "Counter Offset"=w1408, "subtract_mean"=w1407, "downsamp_num"=w1406, "xy_bitshift"=w1405, "x_dg"=w1404, "x_upper_lim"=w1403, "x_lower_lim"=w1402, "x_dc_offset"=w1401, "y_dg"=w1400, "y_upper_lim"=w1399, "y_lower_lim"=w1398, "y_dc_offset"=w1397, "xy_fb_bitshift"=w1396, "z_bitshift"=w1395, "z_set_user"=w1394, "z_pg"=w1393, "z_dg"=w1392, "z_ig"=w1391, "z_fb_bitshift"=w1390, "z_upper_lim"=w1389, "z_lower_lim"=w1388, "z_dc_offset"=w1387, "inject_sigs"=w1378, "downsample->xyz"=w1377, "xy2_bitshift"=w1376, "add_sin"=w1375, "z_internal_inject_freq"=w1374, "z_internal_inject_scale"=w1373, "pow_bitshift"=w1372, "pow_set_user"=w1371, "pow_pg"=w1368, "pow_dg"=w1369, "pow_ig"=w1370, "pow_dc_offset"=w1367, "pow_upper_lim"=w1366, "pow_lower_lim"=w1365, "pow_fb_bitshift"=w1364, "pow_fb"=w1363, "fb_on_pow_set"=w1362, "delta_pow_set_ulim"=w1361, "delta_pow_set_llim"=w1360, "sum_z-pow_fb"=w1359, "subtract_zfb_from_powerr"=w1358, "subtract_zfb_p_scale"=w1356, "subtract_zfb_i_scale"=w1355, "subtract_zfb_d_scale"=w1357, "subtract_zfb_delay"=w1350, "subtract_zfb_ndelay"=w1349, "reset_phi4"=w1351) -> ("FPGA VI Reference Out"=w1353:refnum<k20>, "error out"=w1354:errorcluster)
        n97 = String To Path(string="C:\\Users\\beads\\opt_lev_controls\\labview\\fpga\\fpga_pars") -> (path=w1380:path)
        n98 = case shown="True" w1351 {
          selector: w1351 -> [_ w1414]
          tunnel: w1354 -> [_ w1416]
          tunnel: w1353 -> [_ w1417]
          frame False {
          }
          frame True {
            n99 = flat-sequence {
              tunnel: [w1421] -> w1418
              tunnel: w1417 -> [w1421]
              tunnel: w1416 -> [w1420]
              tunnel: [w1419] -> w1415
              tunnel: w1418 -> [w1425]
              tunnel: w1415 -> [w1424]
              tunnel: w1413 -> [w1423]
              frame #0 {
                n100 = call "Settling Time9"("error in (no error)"=w1420, "Delay Time (s)"=0.001) -> ("error out"=w1419:errorcluster)  [unwired: 9 in]
              }
              frame #1 {
                n101 = xnode "Read/Write Control"("FPGA VI Reference In"=w1425, "error in"=w1424, "reset_phi4"=w1423) -> ()  [unwired: 2 out]
              }
            }
            n102 = Not(x=w1414) -> (.not. x?=w1413:bool)
          }
        }
        n103 = Bundle("phase discont_pos"=w1410, "phase discont_neg"=w1409, "counter offset"=w1408, "subtract_mean"=w1407, "downsamp_num"=w1406, "xy_bitshift"=w1405, "x_dg"=w1404, "x_upper_lim"=w1403, "x_lower_lim"=w1402, "x_dc_offset"=w1401, "y_dg"=w1400, "y_upper_lim"=w1399, "y_lower_lim"=w1398, "y_dc_offset"=w1397, "xy_fb_bitshift"=w1396, "z_bitshift"=w1395, "z_set_init"=w1394, "z_pg"=w1393, "z_dg"=w1392, "z_ig"=w1391, "z_fb_bitshift"=w1390, "z_upper_lim"=w1389, "z_lower_lim"=w1388, "z_off_start"=w1387, "inject_sigs"=w1378, "downsample->xyz"=w1377, "xy2_bitshift"=w1376, "add_sin"=w1375, "z_internal_inject_freq"=w1374, "z_internal_inject_scale"=w1373, "pow_bitshift"=w1372, "pow_set_user"=w1371, "pow_pg"=w1368, "pow_dg"=w1369, "pow_ig"=w1370, "pow_dc_offset"=w1367, "pow_upper_lim"=w1366, "pow_lower_lim"=w1365, "pow_fb_bitshift"=w1364, "pow_fb"=w1363, "fb_on_powset"=w1362, "delta_pow_set_ulim"=w1361, "delta_pow_set_llim"=w1360, "sum_z-pow_fb"=w1359, "subtract_zfb_from_powerr"=w1358, "subtract_zfb_p_scale"=w1356, "subtract_zfb_i_scale"=w1355, "subtract_zfb_d_scale"=w1357, "subtract_zfb_delay"=w1350, "subtract_zfb_ndelay"=w1349) -> (w1352:T4)  [unwired: 1 in]
        n104 = Open/Create/Replace Datalog(5:w1352, 9:enum16{"read/write", "read-only", "write-only"}."read/write" ("access (0:read/write)"), 10:T5."replace or create" ("operation (0:open)"), 11:w1380) -> (0:w1386:errorcluster, 3:w1384:refnum<k1>)  [unwired: 2 in, 1 out]
        n105 = Write Datalog(4:w1386, 6:w1352, 7:w1384) -> (0:w1385:errorcluster, 3:w1383:refnum<k1>)
        n106 = Close File(refnum=w1383, error in=w1385) -> ()  [unwired: 2 out]
      }
    }
    n107 = case shown="True" "Load last pars" {
      tunnel: [w296 w353] -> w93
      tunnel: w94 -> [w296 w353]
      tunnel: [w295 w340] -> w91
      tunnel: w92 -> [w295 w354]
      frame False {
      }
      frame True {
        n108 = String To Path(string="C:\\Users\\beads\\opt_lev_controls\\labview\\fpga\\fpga_pars") -> (path=w357:path)
        n109 = Open/Create/Replace Datalog(5:T4 {"phase discont_pos"=0.0, "phase discont_neg"=0.0, "counter offset"=0, "subtract_mean"=FALSE, "downsamp_num"=0, "xy_bitshift"=0, "x_dg"=0.0, "x_upper_lim"=0, "x_lower_lim"=0, "x_dc_offset"=0, "y_dg"=0.0, "y_upper_lim"=0, "y_lower_lim"=0, "y_dc_offset"=0, "xy_fb_bitshift"=0, "z_bitshift"=0, "z_set_init"=0.0, "z_pg"=0.0, "z_dg"=0.0, "z_ig"=0.0, "z_fb_bitshift"=0, "z_upper_lim"=0, "z_lower_lim"=0, "z_off_start"=0, "inject_sigs"=FALSE, "downsample->xyz"=FALSE, "xy2_bitshift"=0, "add_sin"=FALSE, "z_internal_inject_freq"=0.0, "z_internal_inject_scale"=0, "pow_bitshift"=0, "pow_set_user"=0.0, "pow_pg"=0.0, "pow_dg"=0.0, "pow_ig"=0.0, "pow_dc_offset"=0, "pow_upper_lim"=0, "pow_lower_lim"=0, "pow_fb_bitshift"=0, "pow_fb"=FALSE, "fb_on_powset"=FALSE, "delta_pow_set_ulim"=0.0, "delta_pow_set_llim"=0.0, "sum_z-pow_fb"=FALSE, "subtract_zfb_from_powerr"=FALSE, "subtract_zfb_p_scale"=0.0, "subtract_zfb_i_scale"=0.0, "subtract_zfb_d_scale"=0.0, "subtract_zfb_delay"=FALSE, "subtract_zfb_ndelay"=0} ("output cluster"), 8:w354, 9:enum16{"read/write", "read-only", "write-only"}."read-only" ("access (0:read/write)"), 10:T5."open" ("operation (0:open)"), 11:w357) -> (0:w351:errorcluster, 3:w352:refnum<k1>)  [unwired: 1 in, 1 out]
        n110 = Read Datalog(4:w351, 7:w352) -> (0:w340:errorcluster, 2:w350:T4)  [unwired: 1 in, 1 out]
        n111 = Unbundle(w350) -> ("phase discont_pos"=w349:fxp<+/-,24,12>, "phase discont_neg"=w348:fxp<+/-,24,12>, "counter offset"=w347:u32, "subtract_mean"=w346:bool, "downsamp_num"=w345:i16, "xy_bitshift"=w344:i16, "x_dg"=w343:fxp<+/-,32,16>, "x_upper_lim"=w342:i16, "x_lower_lim"=w341:i16, "x_dc_offset"=w339:i16, "y_dg"=w338:fxp<+/-,32,16>, "y_upper_lim"=w337:i16, "y_lower_lim"=w336:i16, "y_dc_offset"=w335:i16, "xy_fb_bitshift"=w334:i16, "z_bitshift"=w333:i16, "z_set_init"=w332:fxp<+/-,32,32>, "z_pg"=w331:fxp<+/-,32,16>, "z_dg"=w330:fxp<+/-,32,16>, "z_ig"=w329:fxp<+/-,32,16>, "z_fb_bitshift"=w328:i16, "z_upper_lim"=w327:i16, "z_lower_lim"=w326:i16, "z_off_start"=w325:i16, "inject_sigs"=w323:bool, "downsample->xyz"=w322:bool, "xy2_bitshift"=w321:i16, "add_sin"=w320:bool, "z_internal_inject_freq"=w319:fxp<+,32,0>, "z_internal_inject_scale"=w318:i16, "pow_bitshift"=w317:i16, "pow_set_user"=w316:fxp<+/-,32,32>, "pow_pg"=w315:fxp<+/-,32,16>, "pow_dg"=w314:fxp<+/-,32,16>, "pow_ig"=w313:fxp<+/-,32,16>, "pow_dc_offset"=w312:i16, "pow_upper_lim"=w311:i16, "pow_lower_lim"=w310:i16, "pow_fb_bitshift"=w309:i16, "pow_fb"=w308:bool, "fb_on_powset"=w307:bool, "delta_pow_set_ulim"=w306:fxp<+/-,32,32>, "delta_pow_set_llim"=w305:fxp<+/-,32,32>, "sum_z-pow_fb"=w304:bool, "subtract_zfb_from_powerr"=w303:bool, "subtract_zfb_p_scale"=w302:fxp<+/-,32,16>, "subtract_zfb_i_scale"=w301:fxp<+/-,32,16>, "subtract_zfb_d_scale"=w300:fxp<+/-,32,16>, "subtract_zfb_delay"=w298:bool, "subtract_zfb_ndelay"=w297:u8)
        n112 = local write "phase discont_pos"(w349) -> ()
        n113 = local write "phase discont_neg"(w348) -> ()
        n114 = local write "counter offset"(w347) -> ()
        n115 = local write "subtract_mean"(w346) -> ()
        n116 = local write "downsamp_num"(w345) -> ()
        n117 = local write "xy_bitshift"(w344) -> ()
        n118 = local write "x_dg"(w343) -> ()
        n119 = local write "x_upper_lim"(w342) -> ()
        n120 = local write "x_lower_lim"(w341) -> ()
        n121 = local write "x_dc_offset"(w339) -> ()
        n122 = local write "y_dg"(w338) -> ()
        n123 = local write "y_upper_lim"(w337) -> ()
        n124 = local write "y_lower_lim"(w336) -> ()
        n125 = local write "y_dc_offset"(w335) -> ()
        n126 = local write "xy_fb_bitshift"(w334) -> ()
        n127 = local write "z_bitshift"(w333) -> ()
        n128 = local write "z_set_init"(w332) -> ()
        n129 = local write "z_pg"(w331) -> ()
        n130 = local write "z_dg"(w330) -> ()
        n131 = local write "z_ig"(w329) -> ()
        n132 = local write "z_fb_bitshift"(w328) -> ()
        n133 = local write "z_upper_lim"(w327) -> ()
        n134 = local write "z_lower_lim"(w326) -> ()
        n135 = local write "z_dc_offset"(w325) -> ()
        n136 = local write "inject_sigs"(w323) -> ()
        n137 = local write "downsample->xyz"(w322) -> ()
        n138 = local write "xy2_bitshift"(w321) -> ()
        n139 = local write "add_sin"(w320) -> ()
        n140 = local write "z_internal_inject_freq"(w319) -> ()
        n141 = local write "z_internal_inject_scale"(w318) -> ()
        n142 = local write "pow_bitshift"(w317) -> ()
        n143 = local write "pow_set_user"(w316) -> ()
        n144 = local write "pow_pg"(w315) -> ()
        n145 = local write "pow_dg"(w314) -> ()
        n146 = local write "pow_ig"(w313) -> ()
        n147 = local write "pow_dc_offset"(w312) -> ()
        n148 = local write "pow_upper_lim"(w311) -> ()
        n149 = local write "pow_lower_lim"(w310) -> ()
        n150 = local write "pow_fb_bitshift"(w309) -> ()
        n151 = local write "pow_fb"(w308) -> ()
        n152 = local write "fb_on_powset"(w307) -> ()
        n153 = local write "delta_pow_set_ulim"(w306) -> ()
        n154 = local write "delta_pow_set_llim"(w305) -> ()
        n155 = local write "sum_z-pow_fb"(w304) -> ()
        n156 = local write "subtract_zfb_from_powerr"(w303) -> ()
        n157 = local write "subtract_zfb_p_scale"(w302) -> ()
        n158 = local write "subtract_zfb_i_scale"(w301) -> ()
        n159 = local write "subtract_zfb_d_scale"(w300) -> ()
        n160 = local write "subtract_zfb_delay"(w298) -> ()
        n161 = local write "subtract_zfb_ndelay"(w297) -> ()
      }
    }
    n162 = case shown="True" "accept_trigs" {
      selector: "accept_trigs" -> [w382 _]
      tunnel: [w382 w383] -> w60
      tunnel: w91 -> [w380 w387]
      tunnel: w93 -> [w381 w386]
      tunnel: [w381 w385] -> w102
      tunnel: [w380 w384] -> w101
      frame False {
      }
      frame True {
        n163 = xnode "Read/Write Control"("FPGA VI Reference In"=w386, "error in"=w387) -> ("FPGA VI Reference Out"=w385:refnum<k20>, "error out"=w384:errorcluster, "config_trig"=w383:bool)
        "config_trig" <- w383
      }
    }
    n164 = feedback-in #2(w60) -> ()
    n165 = case shown="True" w60 {
      tunnel: w102 -> [w389 w393]
      tunnel: [w389 w400] -> w104
      tunnel: [w388 w399] -> w103
      tunnel: w101 -> [w388 w398]
      tunnel: [w391 w396] -> w73
      tunnel: w72 -> [w391 w397]
      tunnel: w66 -> [w390 w395]
      tunnel: [w390 w394] -> w65
      tunnel: "save_data" -> [_ w392]
      frame False {
      }
      frame True {
        n166 = case shown="True" w392 {
          tunnel: [w403 w462] -> w400
          tunnel: [w404 w461] -> w399
          tunnel: w398 -> [w405 w460]
          tunnel: w397 -> [w402 w459]
          tunnel: [w402 w458] -> w396
          tunnel: w395 -> [w401 w457]
          tunnel: [w401 w456] -> w394
          tunnel: w393 -> [w406 w455]
          frame False {
            n167 = flat-sequence {
              tunnel: [w419] -> w416
              tunnel: w406 -> [w419]
              tunnel: w405 -> [w418]
              tunnel: [w417] -> w415
              tunnel: w416 -> [w423]
              tunnel: w415 -> [w421]
              tunnel: [w422] -> w414
              tunnel: [w420] -> w413
              tunnel: w414 -> [w431]
              tunnel: w413 -> [w430]
              tunnel: [w431] -> w412
              tunnel: [w429] -> w411
              tunnel: w412 -> [w435]
              tunnel: w411 -> [w434]
              tunnel: [w432] -> w410
              tunnel: [w433] -> w409
              tunnel: w410 -> [w439]
              tunnel: w409 -> [w438]
              tunnel: [w439] -> w408
              tunnel: [w437] -> w407
              tunnel: [w440] -> w404
              tunnel: [w441] -> w403
              tunnel: w408 -> [w443]
              tunnel: w407 -> [w442]
              frame #0 {
                n168 = call "Time Delay7"("error in (no error)"=w418) -> ("error out"=w417:errorcluster)  [unwired: 10 in]
              }
              frame #1 {
                w428 = TRUE
                n169 = xnode "Read/Write Control"("FPGA VI Reference In"=w423, "error in"=w421, "block_config_trig"=w428, "TRIG0"=w428) -> ("FPGA VI Reference Out"=w427:refnum<k20>, "error out"=w426:errorcluster)
                n170 = call "config4"("error in (no error)"=w426) -> ("error out"=w425:errorcluster)  [unwired: 10 in]
                n171 = xnode "Read/Write Control"("FPGA VI Reference In"=w427, "error in"=w425, "TRIG0"=FALSE) -> ("FPGA VI Reference Out"=w422:refnum<k20>, "error out"=w420:errorcluster)
              }
              frame #2 {
                n172 = call "Time Delay8"("error in (no error)"=w430) -> ("error out"=w429:errorcluster)  [unwired: 10 in]
              }
              frame #3 {
                n173 = xnode "Read/Write Control"("FPGA VI Reference In"=w435, "error in"=w434, "reset_config_trig"=TRUE) -> ("FPGA VI Reference Out"=w432:refnum<k20>, "error out"=w433:errorcluster)
              }
              frame #4 {
                n174 = call "Time Delay9"("error in (no error)"=w438) -> ("error out"=w437:errorcluster)  [unwired: 10 in]
              }
              frame #5 {
                w444 = FALSE
                n175 = xnode "Read/Write Control"("FPGA VI Reference In"=w443, "error in"=w442, "block_config_trig"=w444, "reset_config_trig"=w444) -> ("FPGA VI Reference Out"=w441:refnum<k20>, "error out"=w440:errorcluster)
              }
            }
          }
          frame True {
            n176 = flat-sequence {
              tunnel: w460 -> [w494]
              tunnel: [w494] -> w492
              tunnel: [w493] -> w491
              tunnel: w455 -> [w493]
              tunnel: [w496] -> w490
              tunnel: w492 -> [w498]
              tunnel: [w495] -> w489
              tunnel: w491 -> [w495]
              tunnel: w490 -> [w527]
              tunnel: [w540] -> w488
              tunnel: [w537] -> w487
              tunnel: [w539] -> w486
              tunnel: [w538] -> w485
              tunnel: w489 -> [w528]
              tunnel: [w529] -> w452
              tunnel: w488 -> [w561]
              tunnel: w487 -> [w562]
              tunnel: [w576] -> w484
              tunnel: [w575] -> w483
              tunnel: [w569] -> w482
              tunnel: [w568] -> w481
              tunnel: [w574] -> w480
              tunnel: w486 -> [w574]
              tunnel: [w573] -> w479
              tunnel: w485 -> [w573]
              tunnel: [w572] -> w478
              tunnel: [w567] -> w477
              tunnel: [w563] -> w453
              tunnel: w452 -> [w563]
              tunnel: [w554] -> w451
              tunnel: [w553] -> w450
              tunnel: [w552] -> w447
              tunnel: w484 -> [w623]
              tunnel: w483 -> [w628]
              tunnel: w482 -> [w627]
              tunnel: w481 -> [w626]
              tunnel: w480 -> [w625]
              tunnel: w479 -> [w624]
              tunnel: [w622] -> w476
              tunnel: w478 -> [w622]
              tunnel: [w621] -> w475
              tunnel: [w620] -> w474
              tunnel: w477 -> [w620]
              tunnel: [w619] -> w473
              tunnel: [w618] -> w472
              tunnel: [w617] -> w471
              tunnel: [w616] -> w470
              tunnel: [w615] -> w469
              tunnel: w453 -> [w606]
              tunnel: w451 -> [w608]
              tunnel: w450 -> [w607]
              tunnel: [w605] -> w449
              tunnel: [w604] -> w448
              tunnel: w447 -> [w604]
              tunnel: [w603] -> w446
              tunnel: [w602] -> w445
              tunnel: w476 -> [w692]
              tunnel: w475 -> [w691]
              tunnel: w474 -> [w690]
              tunnel: w473 -> [w689]
              tunnel: w472 -> [w688]
              tunnel: w471 -> [w687]
              tunnel: w470 -> [w685]
              tunnel: w469 -> [w686]
              tunnel: [w684] -> w468
              tunnel: [w683] -> w467
              tunnel: [w671] -> w454
              tunnel: w449 -> [w664]
              tunnel: w448 -> [w663]
              tunnel: w446 -> [w662]
              tunnel: w445 -> [w661]
              tunnel: w468 -> [w1306]
              tunnel: [w1306] -> w466
              tunnel: w467 -> [w1304]
              tunnel: [w1303] -> w465
              tunnel: w454 -> [w1305]
              tunnel: w466 -> [w1311]
              tunnel: w465 -> [w1310]
              tunnel: [w1309] -> w464
              tunnel: [w1308] -> w463
              tunnel: [w1319] -> w461
              tunnel: [w1320] -> w462
              tunnel: w464 -> [w1320]
              tunnel: w463 -> [w1319]
              tunnel: w459 -> [w1317]
              tunnel: [w1316] -> w458
              tunnel: w457 -> [w1314]
              tunnel: [w1313] -> w456
              frame #0 {
              }
              frame #1 {
                n177 = String To Path(string="C:\\Users\\beads\\opt_lev_controls\\labview\\fpga\\fpga_daq_config") -> (path=w524:path)
                n178 = Open/Create/Replace File(file path (use dialog)=w524, error in=w498, operation (0:open)=T5."open", access (0:read/write)=enum16{"read/write", "read-only", "write-only"}."read-only") -> (refnum out=w521:refnum<file>, error out=w520:errorcluster)  [unwired: 2 in, 1 out]
                n179 = Read from Text File(file (use dialog)=w521, error in=w520) -> (refnum out=w519:refnum<file>, text=w517:string, error out=w518:errorcluster)  [unwired: 2 in, 1 out]
                n180 = Spreadsheet String To Array(delimiter (Tab)="\n", format string="%s", spreadsheet string=w517, array type (2D Dbl)=string[] [] ("array of strings")) -> (array=w513:string[])
                n181 = Close File(refnum=w519, error in=w518) -> (error out=w497:errorcluster)  [unwired: 1 out]
                n182 = Index Array(array=w513) -> (element #1=w512:string, element #2=w509:string, element #3=w501:string)  [unwired: 3 in]
                n183 = String To Path(string=w512) -> (path=w511:path)
                n184 = String Length(string=w509) -> (length=w508:i32)
                n185 = Subtract(x=w508, y=3) -> (x-y=w506:i32)
                n186 = String Subset(string=w509, offset (0)=0, length (rest)=w506) -> (substring=w505:string)
                n187 = Concatenate Strings(w505, "_fpga.h5" ("string")) -> (w503:string)
                n188 = Fract/Exp String To Number(string=w501) -> (number=w500:dbl)  [unwired: 3 in, 1 out]
                n189 = Build Path(base path=w511, name or relative path=w503) -> (appended path=→"fpga_dat_path":path)
                n190 = To Unsigned Long Integer(number=w500) -> (unsigned 32bit integer=→"Nsamp_config":u32)
                n191 = call "Time Delay2"("error in (no error)"=w497) -> ("error out"=w496:errorcluster)  [unwired: 10 in]
              }
              frame #2 {
                w530 = u32 1 ("Extra Samps")
                n192 = local read "Nsamp_config"() -> (w531:u32)
                n193 = Wait (ms)(milliseconds to wait=u32 1) -> ()  [unwired: 1 out]
                n194 = xnode "Invoke Method"("FPGA VI Reference In"=w528, "error in"=w527) -> ("error out"=w526:errorcluster)  [unwired: 1 out]
                n195 = xnode "Invoke Method"("FPGA VI Reference In"=w528, "error in"=w527) -> ("error out"=w542:errorcluster)  [unwired: 1 out]
                n196 = xnode "Invoke Method"("FPGA VI Reference In"=w528, "error in"=w527) -> ("FPGA VI Reference Out"=w537:refnum<k20>, "error out"=w541:errorcluster)
                n197 = Multiply(x=w531, y=u32 12) -> (x*y=w544:u32)
                n198 = Multiply(x=w531, y=u32 4) -> (x*y=w532:u32)
                n199 = Multiply(x=w531, y=u32 11) -> (x*y=w543:u32)
                n200 = Quotient & Remainder(x=w532, y=u32 8190) -> (floor(x/y)=w534:u32)  [unwired: 1 out]
                n201 = Quotient & Remainder(x=w543, y=u32 8190) -> (floor(x/y)=w546:u32)  [unwired: 1 out]
                n202 = Quotient & Remainder(x=w544, y=u32 8190) -> (floor(x/y)=w548:u32)  [unwired: 1 out]
                n203 = Add(x=w530, y=w534) -> (x+y=w529:u32)
                n204 = Add(x=w530, y=w548) -> (x+y=w539:u32)
                n205 = Add(x=w530, y=w546) -> (x+y=w538:u32)
                n206 = Merge Errors(w541, w542, w526) -> (w540:errorcluster)
                "config_loaded" <- TRUE
              }
              frame #3 {
                w558 = -1 ("Timeout (ms)")
                w559 = u32 0 ("Elements Remaining")
                w560 = -1
                # "Start reading out data waiting for the start trig from DAQ"
                # "Clear all the data in the FIFOs"
                n207 = while {
                  tunnel: w560 -> [w596]
                  shift-right: [w598] -> w577
                  shift-left: w562 -> [w601]
                  shift-right: [w597] -> w566
                  shift-left: w561 -> [w600]
                  shift-right: [w595] -> _
                  shift-left: w559 -> [w599]
                  stop <- w594 stop-if-true
                  n208 = xnode "Invoke Method"("FPGA VI Reference In"=w601, "error in"=w600, "Number of Elements"=w599, "Timeout (ms)"=w596) -> ("FPGA VI Reference Out"=w598:refnum<k20>, "error out"=w597:errorcluster, "Elements Remaining"=w595:u32)  [unwired: 1 out]
                  n209 = Equal To 0?(x=w595) -> (x = 0?=w594:bool)
                }
                n210 = while {
                  tunnel: w560 -> [w583]
                  shift-right: [w580] -> _
                  shift-left: w559 -> [w582]
                  shift-right: [w579] -> w557
                  shift-left: w562 -> [w585]
                  shift-right: [w578] -> w556
                  shift-left: w561 -> [w584]
                  stop <- w581 stop-if-true
                  n211 = xnode "Invoke Method"("FPGA VI Reference In"=w585, "error in"=w584, "Number of Elements"=w582, "Timeout (ms)"=w583) -> ("FPGA VI Reference Out"=w579:refnum<k20>, "error out"=w578:errorcluster, "Elements Remaining"=w580:u32)  [unwired: 1 out]
                  n212 = Equal To 0?(x=w580) -> (x = 0?=w581:bool)
                }
                n213 = while {
                  tunnel: w560 -> [w588]
                  shift-right: [w590] -> w571
                  shift-left: w562 -> [w593]
                  shift-right: [w589] -> w570
                  shift-left: w561 -> [w592]
                  shift-right: [w587] -> _
                  shift-left: w559 -> [w591]
                  stop <- w586 stop-if-true
                  n214 = xnode "Invoke Method"("FPGA VI Reference In"=w593, "error in"=w592, "Number of Elements"=w591, "Timeout (ms)"=w588) -> ("FPGA VI Reference Out"=w590:refnum<k20>, "error out"=w589:errorcluster, "Elements Remaining"=w587:u32)  [unwired: 1 out]
                  n215 = Equal To 0?(x=w587) -> (x = 0?=w586:bool)
                }
                n216 = xnode "Invoke Method"("FPGA VI Reference In"=w577, "error in"=w566, "Number of Elements"=u32 7200, "Timeout (ms)"=w558) -> ("FPGA VI Reference Out"=w576:refnum<k20>, "error out"=w575:errorcluster, "Data"=w572:i32[])  [unwired: 1 out]
                n217 = xnode "Invoke Method"("FPGA VI Reference In"=w571, "error in"=w570, "Number of Elements"=u32 6600, "Timeout (ms)"=w558) -> ("FPGA VI Reference Out"=w569:refnum<k20>, "error out"=w568:errorcluster, "Data"=w567:i32[])  [unwired: 1 out]
                n218 = xnode "Invoke Method"("FPGA VI Reference In"=w557, "error in"=w556, "Number of Elements"=u32 2400, "Timeout (ms)"=w558) -> ("FPGA VI Reference Out"=w554:refnum<k20>, "error out"=w553:errorcluster, "Data"=w552:i32[])  [unwired: 1 out]
              }
              frame #4 {
                w613 = TRUE
                n219 = xnode "Read/Write Control"("FPGA VI Reference In"=w623, "block_config_trig"=w613, "TRIG0"=w613) -> ("FPGA VI Reference Out"=w612:refnum<k20>, "error out"=w611:errorcluster)  [unwired: 1 in]
                n220 = while {
                  shift-right: [w644] -> w616
                  shift-left: w627 -> [w648]
                  shift-right: [w643] -> w615
                  shift-left: w626 -> [w647]
                  tunnel: w624 -> [w640]
                  tunnel: [w639] -> w619 mode=concatenating
                  i -> [w642]
                  stop <- w641 stop-if-true
                  n221 = xnode "Invoke Method"("FPGA VI Reference In"=w648, "error in"=w647, "Number of Elements"=u32 8190, "Timeout (ms)"=-1) -> ("FPGA VI Reference Out"=w644:refnum<k20>, "error out"=w643:errorcluster, "Data"=w639:i32[])  [unwired: 1 out]
                  n222 = Greater?(x=w642, y=w640) -> (0:w641:bool)
                }
                n223 = local write "config_loaded"(FALSE) -> ()
                n224 = while {
                  shift-right: [w654] -> w618
                  shift-left: w623 -> [w658]
                  shift-right: [w653] -> w617
                  shift-left: w628 -> [w657]
                  tunnel: w625 -> [w650]
                  tunnel: [w649] -> w621 mode=concatenating
                  i -> [w652]
                  stop <- w651 stop-if-true
                  n225 = xnode "Invoke Method"("FPGA VI Reference In"=w658, "error in"=w657, "Number of Elements"=u32 8190, "Timeout (ms)"=-1) -> ("FPGA VI Reference Out"=w654:refnum<k20>, "error out"=w653:errorcluster, "Data"=w649:i32[])  [unwired: 1 out]
                  n226 = Greater?(x=w652, y=w650) -> (0:w651:bool)
                }
                n227 = while {
                  tunnel: w606 -> [w632]
                  shift-right: [w631] -> w603
                  shift-left: w608 -> [w638]
                  shift-right: [w630] -> w602
                  shift-left: w607 -> [w637]
                  tunnel: [w629] -> w605 mode=concatenating
                  i -> [w634]
                  stop <- w633 stop-if-true
                  n228 = xnode "Invoke Method"("FPGA VI Reference In"=w638, "error in"=w637, "Number of Elements"=u32 8190, "Timeout (ms)"=-1) -> ("FPGA VI Reference Out"=w631:refnum<k20>, "error out"=w630:errorcluster, "Data"=w629:i32[])  [unwired: 1 out]
                  n229 = Greater?(x=w634, y=w632) -> (0:w633:bool)
                }
                n230 = call "config"("error in (no error)"=w611) -> ("error out"=w610:errorcluster)  [unwired: 10 in]
                n231 = xnode "Read/Write Control"("FPGA VI Reference In"=w612, "error in"=w610, "TRIG0"=FALSE) -> ()  [unwired: 2 out]
              }
              frame #5 {
                w665 = LVH5D_Operation."create or replace" ("operation (open or create)")
                n232 = Build Array (concatenate)(w692, w691) -> (w679:i32[])
                n233 = Build Array (concatenate)(w690, w689) -> (w674:i32[])
                n234 = local read "fpga_dat_path"() -> (w681:path)
                n235 = Build Array (concatenate)(w663, w664) -> (w659:i32[])
                n236 = call <vilib>:"OpenCreateReplace HDF5 File.vi"("function (open or create)"=LVH5F_Operation."create or replace", "path"=w681) -> ("error out"=w672:errorcluster, "HDF5 Ref out"=w673:T12)  [unwired: 6 in]
                n237 = xnode "Invoke Method"("FPGA VI Reference In"=w688, "error in"=w687) -> ("FPGA VI Reference Out"=w694:refnum<k20>, "error out"=w696:errorcluster)
                n238 = xnode "Invoke Method"("FPGA VI Reference In"=w685, "error in"=w686) -> ("error out"=w695:errorcluster)  [unwired: 1 out]
                n239 = xnode "Invoke Method"("FPGA VI Reference In"=w662, "error in"=w661) -> ("error out"=w660:errorcluster)  [unwired: 1 out]
                n240 = xnode "Simple H5Dwrite"("Dataset Path"="beads/data/quad_data" ("dataset name"), "error in (no error)"=w672, "operation (open or create)"=w665, "HDF5 Path or Ref"=w673, "Data"=w679) -> ("HDF5 Ref out"=w677:T12, "error out"=w676:errorcluster)  [unwired: 3 in, 1 out]
                n241 = xnode "Simple H5Dwrite"("Dataset Path"="beads/data/pos_data" ("dataset name"), "error in (no error)"=w676, "operation (open or create)"=w665, "HDF5 Path or Ref"=w677, "Data"=w674) -> ("HDF5 Ref out"=w670:T12, "error out"=w669:errorcluster)  [unwired: 3 in, 1 out]
                n242 = Merge Errors(w696, w695, w660) -> (w682:errorcluster)
                n243 = xnode "Simple H5Dwrite"("Dataset Path"="beads/data/pow_data" ("dataset name"), "error in (no error)"=w669, "operation (open or create)"=w665, "HDF5 Path or Ref"=w670, "Data"=w659) -> ("HDF5 Ref out"=w667:T12, "error out"=w668:errorcluster)  [unwired: 3 in, 1 out]
                n244 = xnode "Read/Write Control"("FPGA VI Reference In"=w694, "error in"=w682, "reset_config_trig"=TRUE) -> ("FPGA VI Reference Out"=w684:refnum<k20>, "error out"=w683:errorcluster)
                n245 = call <vilib>:"H5Fclose.vi"("error in (no error)"=w668, "HDF5 Ref"=w667) -> ("error out"=w671:errorcluster)  [unwired: 7 in]
              }
              frame #6 {
                n246 = call "Time Delay3"() -> ()  [unwired: 11 in, 1 out]
                n247 = Merge Errors(w1305, w1304) -> (w1303:errorcluster)
              }
              frame #7 {
                w1307 = FALSE
                n248 = xnode "Read/Write Control"("FPGA VI Reference In"=w1311, "error in"=w1310, "block_config_trig"=w1307, "reset_config_trig"=w1307) -> ("FPGA VI Reference Out"=w1309:refnum<k20>, "error out"=w1308:errorcluster)
              }
              frame #8 {
                n249 = local read "step_z_offset"() -> (w1315:bool)
                n250 = case shown="True" w1315 {
                  tunnel: w1314 -> [w1321 w1324]
                  tunnel: [w1321 w1322] -> w1313
                  tunnel: "z_off_step" -> [_ w1323]
                  frame False {
                  }
                  frame True {
                    n251 = Add(x=w1324, y=w1323) -> (x+y=w1322:i16)
                  }
                }
                n252 = case shown="True" "step_z_set" {
                  tunnel: [w1325 w1327] -> w1316
                  tunnel: w1317 -> [w1325 w1326]
                  frame False {
                  }
                  frame True {
                    n253 = Add(x=w1326, y="z_set_step") -> (x+y=w1327:fxp<+/-,32,32>)
                  }
                }
              }
            }
          }
        }
      }
    }
    n254 = case shown="False" "show_quad" {
      tunnel: [w267 w294] -> w162
      tunnel: [w266 w293] -> w161
      tunnel: [w265 w292] -> w159
      tunnel: [w258 w291] -> w158
      tunnel: [w258 w290] -> w157
      tunnel: [w258 w289] -> w156
      tunnel: [w258 w288] -> w155
      tunnel: [w264 w287] -> w135
      tunnel: [w263 w286] -> w134
      tunnel: [w262 w285] -> w133
      tunnel: [w261 w284] -> w132
      tunnel: [w260 w283] -> w131
      tunnel: [w259 w282] -> w130
      tunnel: [w258 w281] -> w112
      tunnel: [w258 w280] -> w111
      tunnel: w104 -> [w269 w279]
      tunnel: w103 -> [w268 w278]
      tunnel: [w258 w277] -> w86
      tunnel: [w258 w276] -> w85
      tunnel: [w258 w275] -> w84
      tunnel: [w258 w274] -> w83
      tunnel: [w257 w273] -> w61
      tunnel: [w256 w272] -> w42
      tunnel: [w254 w271] -> w24
      tunnel: [w255 w270] -> w23
      frame False {
        w258 = fxp<+/-,32,18> 0.0 ("phi0_full_out")
        n255 = xnode "Read/Write Control"("FPGA VI Reference In"=w269, "error in"=w268) -> ("FPGA VI Reference Out"=w267:refnum<k20>, "error out"=w266:errorcluster, "loop time"=w265:fxp<+,32,32>, "x_shifted"=w264:i32, "x_fb_i16"=w263:i16, "y_shifted"=w262:i32, "y_fb_i16"=w261:i16, "z_shifted"=w260:i32, "z_fb_i16"=w259:i16, "z_fb_tot_i16"=w257:i16, "pow_shifted"=w256:i32, "pow_fb_i16"=w255:i16, "delta_pow_set"=w254:fxp<+/-,32,32>)
      }
      frame True {
        n256 = xnode "Read/Write Control"("FPGA VI Reference In"=w279, "error in"=w278) -> ("FPGA VI Reference Out"=w294:refnum<k20>, "error out"=w293:errorcluster, "phi0_full_out"=w274:fxp<+/-,32,18>, "phi1_full_out"=w277:fxp<+/-,32,18>, "phi2_full_out"=w276:fxp<+/-,32,18>, "phi3_full_out"=w275:fxp<+/-,32,18>, "phi4_full_out"=w281:fxp<+/-,32,18>, "amp0_out"=w288:fxp<+,32,16>, "amp1_out"=w289:fxp<+,32,16>, "amp2_out"=w290:fxp<+,32,16>, "amp3_out"=w291:fxp<+,32,16>, "amp4_out"=w280:fxp<+,32,16>, "loop time"=w292:fxp<+,32,32>, "x_shifted"=w287:i32, "x_fb_i16"=w286:i16, "y_shifted"=w285:i32, "y_fb_i16"=w284:i16, "z_shifted"=w283:i32, "z_fb_i16"=w282:i16, "z_fb_tot_i16"=w273:i16, "pow_shifted"=w272:i32, "pow_fb_i16"=w270:i16, "delta_pow_set"=w271:fxp<+/-,32,32>)
      }
    }
    "phi1" <- w86
    "phi0" <- w83
    "loop time" <- w159
    "phi3" <- w84
    "phi2" <- w85
    "amp1" <- w156
    "amp0" <- w155
    "amp3" <- w158
    "amp2" <- w157
    "x" <- w135
    "x_fb" <- w134
    "y" <- w133
    "y_fb" <- w132
    "z" <- w131
    "z_fb" <- w130
    "phi4" <- w112
    "amp4" <- w111
    "z_fb_tot" <- w61
    "delta_pow_set" <- w24
    "pow" <- w42
    "pow_fb" <- w23
    n257 = Subtract(x=w83, y=w83) -> (x-y=w82:fxp<+/-,33,19>)
    n258 = Subtract(x=w86, y=w83) -> (x-y=w81:fxp<+/-,33,19>)
    n259 = Subtract(x=w85, y=w83) -> (x-y=w80:fxp<+/-,33,19>)
    n260 = Subtract(x=w84, y=w83) -> (x-y=w79:fxp<+/-,33,19>)
    n261 = Bundle(w82, w81, w80, w79) -> (→"delta_phi":T13)  [unwired: 1 in]
  }
  n262 = xnode "Close FPGA VI Reference"("FPGA VI Reference In"=w14, "error in"=w13) -> ("error out"=w15:errorcluster)
  n263 = call <vilib>:"Simple Error Handler.vi"("error in (no error)"=w15) -> ()  [unwired: 4 in, 5 out]
